vi "Arduino_comms_Global.vi"() -> ()   [LabVIEW 2012]
uses:
  Arduino_comm_params.ctl
panel:
  in  "Arduino comm. params.":T1={"VISA resource name"="COM9", "byte count"=64, "flow control (0:none)"=0, "stop bits (10: 1 bit)"=10, "parity (0:none)"=enum."None", "data bits (8)"=8, "termination char "=10, "Enable Termination\nChar"=TRUE, "baud rate (bps)"=115200, "timeout (ms)"=10000, "Locked"=FALSE} {"termination char" format="%02x"; "data bits (8)" min=5 max=8 step=1; "stop bits (10: 1 bit)" items=["1.0"=10, "1.5"=15, "2.0"=20]; "flow control (0:none)" items=["None", "XON/XOFF", "RTS/CTS", "XON/XOFF & RTS/CTS", "DTR/DSR", "XON/XOFF & DTR/DSR"]}
  # "(0xA = '\\n' = newline)"
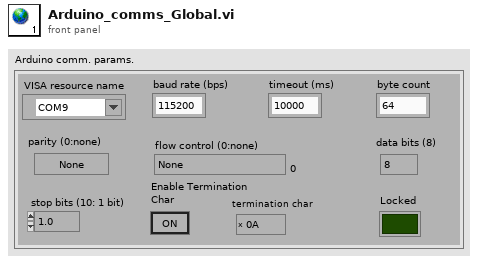
[diagram p1: front panel]
types:
  T1 = typedef "Arduino_comm_params.ctl" = cluster{"VISA resource name":refnum<visa-resource-name>, "byte count":u32, "flow control (0:none)":u16, "stop bits (10: 1 bit)":u16, "parity (0:none)":enum16{"None", "Odd", "Even", "Mark", "Space"}, "data bits (8)":u16, "termination char ":u8, "Enable Termination\nChar":bool, "baud rate (bps)":u32, "timeout (ms)":u32, "Locked":bool}
diagram:
